vi "WPI_CameraGet Color Level.vi"(8 "error in (no error)":errorcluster, 11 "CameraDevRef":T1={"Camera Address"="192.168.0.90", "CameraStatus"={"status"=FALSE, "code"=0, "source"=""}}) -> (0 "error out":errorcluster, 2 "Color Level":i32, 3 "CameraDevRef Out":T1)   [LabVIEW 2017]
doc: "Returns the color level setting of the camera you specify.\n\nThis software is licensed. Open the labview\\readme\\WPI Robotics Library Open Source License.txt file for more information."
uses:
  <vilib>/Rock Robotics/WPI/Camera/WPI_CameraDevRef.ctl
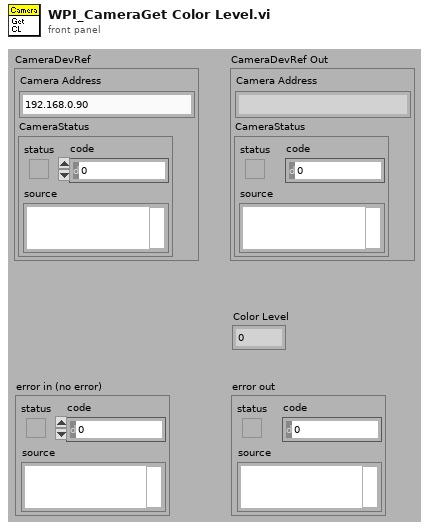
[diagram p1: front panel]
types:
  T1 = typedef "WPI_CameraDevRef.ctl" = cluster{"Camera Address":string, "CameraStatus":errorcluster}
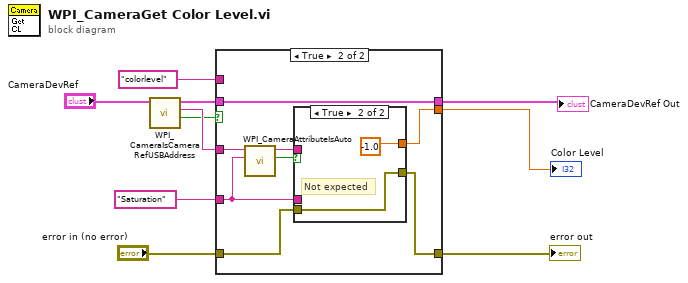
[diagram p0: block diagram]
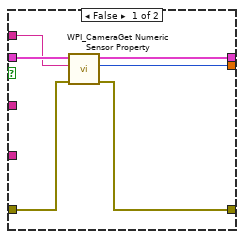
[diagram p2: hidden frame]
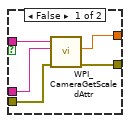
[diagram p3: hidden frame]
diagram:
  n1 = call <vilib>:"WPI_CameraIsCameraRefUSBAddress.vi"("CameraDevRef"="CameraDevRef") -> ("USB?"=w3:bool, "Camera Address Out"=w4:string, "CameraDevRef out"=w1:T1)  [unwired: 7 in, 1 out]
  n2 = case shown="True" w3 {
    tunnel: w1 -> [w16 w19]
    tunnel: [w15 w19] -> w10
    tunnel: "colorlevel" ("Property Name") -> [w14 _]
    tunnel: [w13 w20] -> w8
    tunnel: "error in (no error)" -> [w12 w18]
    tunnel: [w11 w17] -> w6
    tunnel: w4 -> [_ w24]
    tunnel: "Saturation" -> [_ w23]
    frame False {
      n3 = call <vilib>:"WPI_CameraGet Numeric Sensor Property.vi"("error in (no error)"=w12, "Property Name"=w14, "CameraDevRef"=w16) -> ("error out"=w11:errorcluster, "Value"=w13:i32, "CameraDevRef dup"=w15:T1)  [unwired: 2 in, 4 out]
    }
    frame True {
      n4 = call <vilib>:"WPI_CameraAttributeIsAuto.vi"("Attr String"=w23, "Camera Address In"=w24) -> ("Auto?"=w21:bool, "Camera Address Out"=w22:string)  [unwired: 8 in]
      n5 = case shown="True" w21 {
        tunnel: w23 -> [w28 _]
        tunnel: w22 -> [w29 _]
        tunnel: [w27 -1.0] -> w20
        tunnel: w18 -> [w26 w30]
        tunnel: [w25 w30] -> w17
        frame False {
          n6 = call <vilib>:"WPI_CameraGetScaledAttr.vi"("error in (no error)"=w26, "Attr String"=w28, "Camera Address In"=w29) -> ("error out"=w25:errorcluster, "Scaled"=w27:dbl)  [unwired: 5 in, 2 out]
        }
        frame True {
          # "Not expected"
        }
      }
    }
  }
  "CameraDevRef Out" <- w10
  "Color Level" <- w8
  "error out" <- w6
